vi "Write Raw Data Network Stream.vi"(8 "error in (no error)":errorcluster) -> (0 "error out":errorcluster)   [LabVIEW 2017]
uses:
  RTLSDR Control/RTLSDR Global Variables.vi
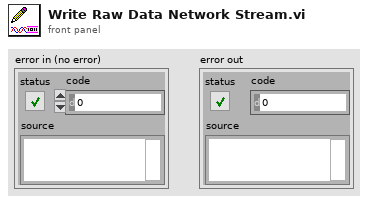
[diagram p1: front panel]
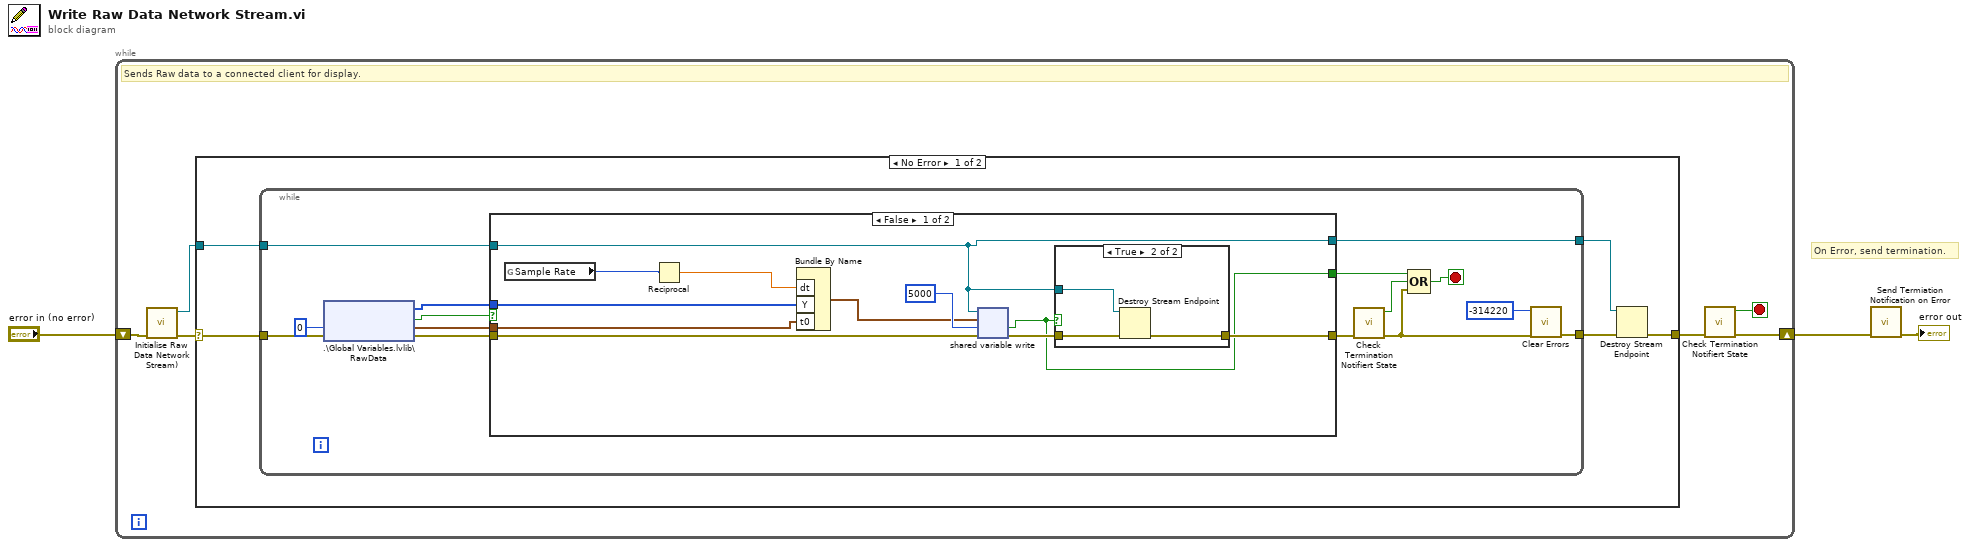
[diagram p0: block diagram]
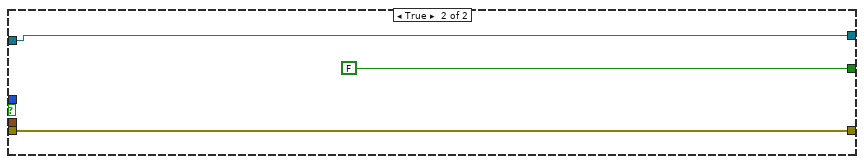
[diagram p3: hidden frame]
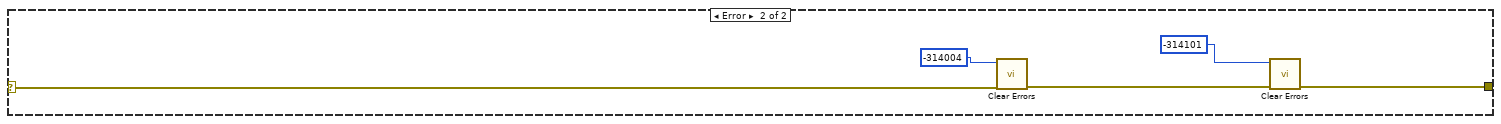
[diagram p4: hidden frame]
diagram:
  # "On Error, send termination."
  n1 = while {
    shift-right: [w7] -> w2
    shift-left: "error in (no error)" -> [w5]
    stop <- w9 stop-if-true
    # "Sends Raw data to a connected client for display."
    n2 = call "Initialise Raw Data Network Stream).vi"("error in (no error)"=w5) -> ("error out"=w6:errorcluster, "Refnum out"=w4:refnum<k21>)  [unwired: 9 in]
    n3 = case shown="No Error" w6 {
      selector: w6 -> [w14 w49]
      tunnel: [w12 w52] -> w8
      tunnel: w4 -> [w11 _]
      frame No Error {
        n4 = while {
          tunnel: w14 -> [w20]
          tunnel: [w26] -> w13
          tunnel: w11 -> [w22]
          tunnel: [w21] -> w10
          stop <- w27 stop-if-true
          n5 = shared-variable ".\\Global Variables.lvlib\\RawData"(error in=w20, 0 ("ms timeout (0)")) -> (w18:u8[], error out=w19:errorcluster, w17:bool, w15:timestamp)
          n6 = case shown="False" w17 {
            tunnel: w19 -> [w40 w46]
            tunnel: w18 -> [w31 _]
            tunnel: [w38 w46] -> w29
            tunnel: [w37 FALSE] -> w23
            tunnel: w22 -> [w35 w45]
            tunnel: [w35 w45] -> w21
            tunnel: w15 -> [w30 _]
            frame False {
              n7 = global read "RTLSDR Global Variables.vi" "Sample Rate"() -> (w33:u32)
              n8 = Reciprocal(x=w33) -> (1/x=w32:dbl)
              n9 = Bundle By Name("dt"=w32, "Y"=w31, "t0"=w30) -> (w34:waveform(u8))  [unwired: 1 in]
              n10 = shared-variable-write(w35, w40, w34, 5000 ("timeout ms (-1)")) -> (w39:errorcluster, w37:bool)  [unwired: 1 out]
              n11 = case shown="True" w37 {
                tunnel: w39 -> [w41 w44]
                tunnel: [w41 w43] -> w38
                tunnel: w35 -> [_ w42]
                frame False {
                }
                frame True {
                  n12 = Destroy Stream Endpoint(8:w44, 11:w42) -> (0:w43:errorcluster)
                }
              }
            }
            frame True {
            }
          }
          n13 = call "Check Termination Notifiert State.vi"("error in (no error)"=w29) -> ("error out"=w24:errorcluster, "Termination Notifier State"=w28:bool)  [unwired: 9 in]
          n14 = Compound Arithmetic op=OR(w23, w28, w24) -> (w27:bool)
          n15 = call <vilib>:"Clear Errors.vi"("error in (no error)"=w24, "specific error code to clear (0: all)"=-314220) -> ("error out"=w26:errorcluster)  [unwired: 4 in, 1 out]
        }
        n16 = Destroy Stream Endpoint(8:w13, 11:w10) -> (0:w12:errorcluster)
      }
      frame Error {
        n17 = call <vilib>:"Clear Errors.vi"("error in (no error)"=w49, "specific error code to clear (0: all)"=-314004 ("y")) -> ("error out"=w50:errorcluster)  [unwired: 4 in, 1 out]
        n18 = call <vilib>:"Clear Errors.vi"("error in (no error)"=w50, "specific error code to clear (0: all)"=-314101) -> ("error out"=w52:errorcluster)  [unwired: 4 in, 1 out]
      }
    }
    n19 = call "Check Termination Notifiert State.vi"("error in (no error)"=w8) -> ("error out"=w7:errorcluster, "Termination Notifier State"=w9:bool)  [unwired: 9 in]
  }
  n20 = call "Send Termiation Notification on Error.vi"("error in (no error)"=w2) -> ("error out"=→"error out":errorcluster)  [unwired: 10 in]
